vi "v2mv.vi"(4 "error in":errorcluster, 5 "ArrayIn":waveform(dbl)[](array[waveform])) -> (0 "error out":errorcluster, 1 "ArrayOut":waveform(i16)[](array[waveform]), 2 "t0":timestamp)   [LabVIEW 2010]
uses:
  lib/Global 2.vi
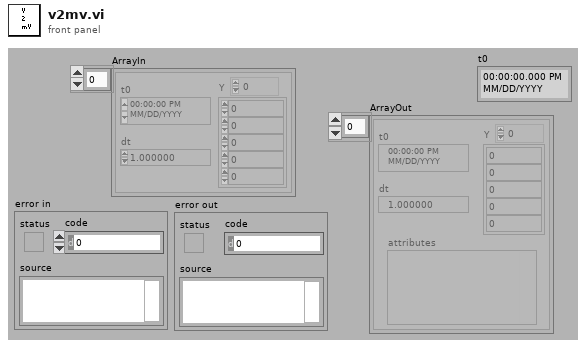
[diagram p1: front panel]
types:
  T1 = cluster{"name":enum16{"sync", "phase_a", "phase_b", "phase_c", "ground"}, "num":i32}[]
  T2 = enum16{"sync", "phase_a", "phase_b", "phase_c", "ground"}
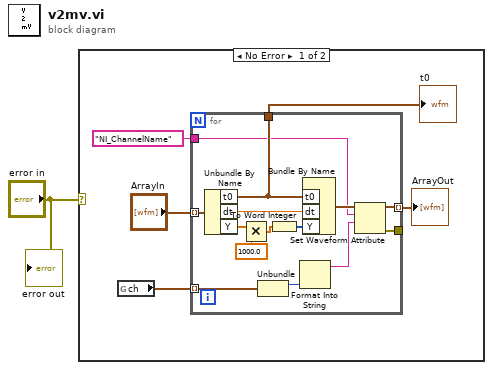
[diagram p0: block diagram]
diagram:
  n1 = case shown="No Error" "error in" {
    frame No Error {
      n2 = global read "Global 2.vi" "ch"() -> (w2:T1)
      n3 = for {
        tunnel: "ArrayIn" -> [w20] mode=indexing
        tunnel: [w16] -> w6
        tunnel: "NI_ChannelName" ("name") -> [w12]
        tunnel: [w11] -> _
        tunnel: [w10] -> w3 mode=indexing
        tunnel: w2 -> [w8] mode=indexing
        n4 = Unbundle By Name(w20) -> ("t0"=w16:timestamp, "dt"=w15:dbl, "Y"=w19:dbl[])
        n5 = Multiply(x=w19, y=1000.0) -> (x*y=w18:dbl[])
        n6 = Unbundle(w8) -> ("name"=w7:T2)  [unwired: 1 out]
        n7 = To Word Integer(number=w18) -> (16bit integer=w14:i16[])
        n8 = Format Into String(w7) -> (resulting string=w9:string)  [unwired: 3 in, 1 out]
        n9 = Bundle By Name("t0"=w16, "dt"=w15, "Y"=w14) -> (w13:waveform(i16))  [unwired: 1 in]
        n10 = Set Waveform Attribute(5:w9, 6:w12, 7:w13) -> (0:w11:errorcluster, 3:w10:waveform(i16))  [unwired: 1 in, 1 out]
      }
      "t0" <- w6
      "ArrayOut" <- w3
    }
    frame Error {
    }
  }
  "error out" <- "error in"
